vi "find_peaks.vi"(10 "ranges":T1(array[cluster])=[{"min"=0.0, "max"=1000.0, "Sensibilidade"=50.0}] caption="Faixas" {"Sensibilidade" min=0.0 max=100.0 format="%#_g %"; "max" min=0.0 format="%#_g Hz"; "min" min=0.0 format="%#_g Hz"}, 11 "data":cluster{"freqs":dbl[], "Array":dbl[]}[](array[cluster])) -> (1 "#freqs":i32[](array[numeric]), 2 "freqs":dbl[][](array[numeric]), 3 "plots":cluster{"Array":dbl[], "Array":dbl[]}[](array[cluster]))   [LabVIEW 2016]
uses:
  <vilib>/Analysis/NI_AAL_SigProc.lvlib
  <vilib>/gmath/NI_Gmath.lvlib
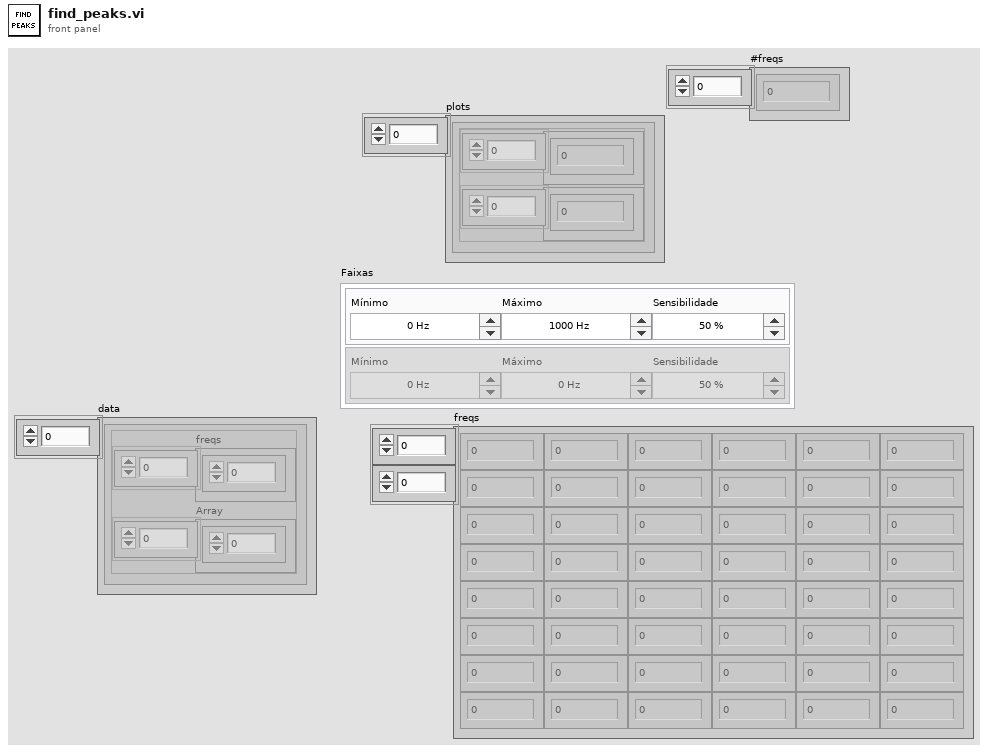
[diagram p1: front panel]
types:
  T1 = cluster{"min":dbl, "max":dbl, "Sensibilidade":dbl}[]
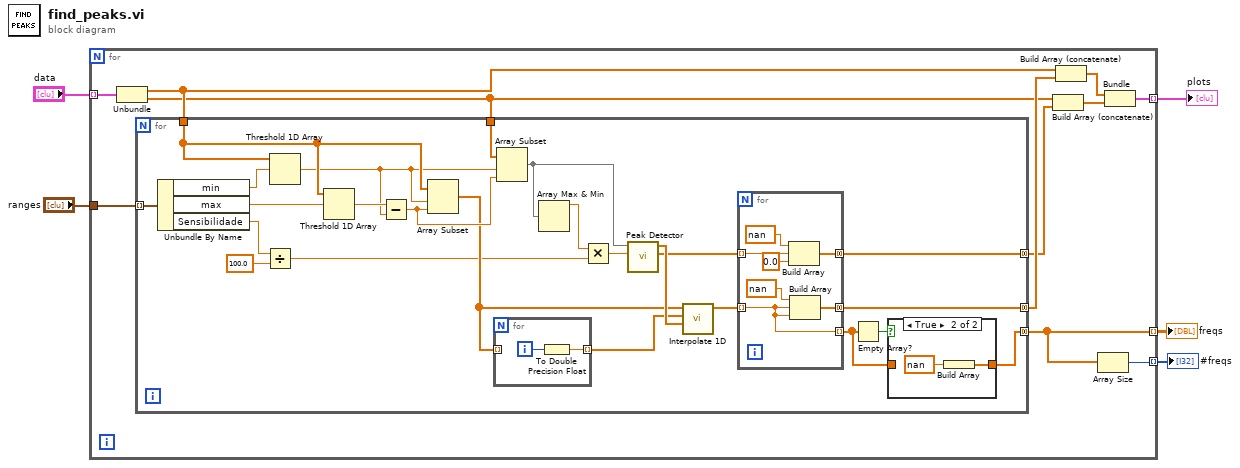
[diagram p0: block diagram]
diagram:
  n1 = for {
    tunnel: "data" -> [w16] mode=indexing
    tunnel: "ranges" -> [w15]
    tunnel: [w10] -> w4 mode=indexing
    tunnel: [w7] -> w2 mode=indexing
    tunnel: [w6] -> w1 mode=indexing
    n2 = Unbundle(w16) -> ("freqs"=w9:dbl[], "Array"=w8:dbl[])
    n3 = for {
      tunnel: w9 -> [w36]
      tunnel: w15 -> [w40] mode=indexing
      tunnel: w8 -> [w34]
      tunnel: [w24] -> w11 mode=concatenating
      tunnel: [w23] -> w12 mode=concatenating
      tunnel: [w18] -> w7 mode=concatenating
      n4 = Unbundle By Name(w40) -> ("min"=w39:dbl, "max"=w38:dbl, "Sensibilidade"=w21:dbl)
      n5 = Divide(x=w21, y=100.0) -> (x/y=w20:dbl)
      n6 = Threshold 1D Array(2:w39, 3:w36) -> (0:w35:dbl)  [unwired: 1 in]
      n7 = Threshold 1D Array(2:w38, 3:w36) -> (0:w37:dbl)  [unwired: 1 in]
      n8 = Subtract(x=w37, y=w35) -> (x-y=w33:dbl)
      n9 = Array Subset(array=w36, index=w35, length=w33) -> (w28:dbl[])
      n10 = for {
        tunnel: w28 -> [_] mode=indexing
        tunnel: [w52] -> w27 mode=indexing
        i -> [w51]
        n11 = To Double Precision Float(number=w51) -> (double precision float=w52:dbl)
      }
      n12 = Array Subset(array=w34, index=w35, length=w33) -> (w30:dbl[])
      n13 = Array Max & Min(array=w30) -> (max value=w32:dbl)  [unwired: 3 out]
      n14 = Multiply(x=w32, y=w20) -> (x*y=w31:dbl)
      n15 = call <vilib>:"Peak Detector.vi"("threshold"=w31, "X"=w30) -> ("Amplitudes"=w25:dbl[], "Locations"=w29:dbl[])  [unwired: 5 in, 3 out]
      n16 = call <vilib>:"Interpolate 1D.vi"("xi"=w29, "X"=w27, "Y"=w28) -> ("yi"=w26:dbl[])  [unwired: 6 in, 2 out]
      n17 = for {
        tunnel: w26 -> [w44] mode=indexing
        tunnel: w25 -> [w50] mode=indexing
        tunnel: [w47] -> w23 mode=concatenating
        tunnel: [w46] -> w24 mode=concatenating
        tunnel: [w44] -> w17 mode=indexing
        n18 = Build Array(nan ("element"), w50, 0.0 ("element")) -> (w46:dbl[])
        n19 = Build Array(nan ("element"), w44, w44) -> (w47:dbl[])
      }
      n20 = Empty Array?(array=w17) -> (empty?=w19:bool)
      n21 = case shown="True" w19 {
        tunnel: [w41 w42] -> w18
        tunnel: w17 -> [w41 _]
        frame False {
        }
        frame True {
          n22 = Build Array(nan ("element")) -> (w42:dbl[])
        }
      }
    }
    n23 = Build Array (concatenate)(w8, w11) -> (w13:dbl[])
    n24 = Build Array (concatenate)(w9, w12) -> (w14:dbl[])
    n25 = Array Size(array=w7) -> (size(s)=w6:i32)
    n26 = Bundle(w14, w13) -> (w10:cluster{dbl[], dbl[]})  [unwired: 1 in]
  }
  "plots" <- w4
  "freqs" <- w2
  "#freqs" <- w1
